vi "Add data or replace.vi"(9 "Power data":cluster{"Frequency (GHz)":dbl, "Power (mW)":dbl}, 10 "Index":i32, 11 "Power readings in":cluster{"Frequency":dbl, "Power":dbl}[](array[cluster])) -> (3 "Power readings out":cluster{"Frequency":dbl, "Power":dbl}[](array[cluster]))   [LabVIEW 2019, in "Power control.lvclass"]
uses:
  Power control.lvclass
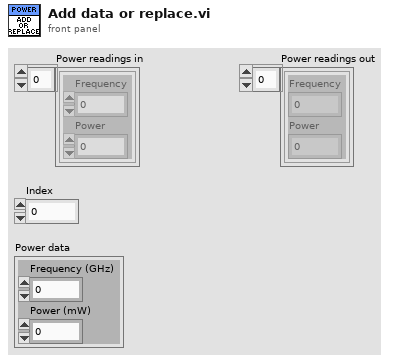
[diagram p1: front panel]
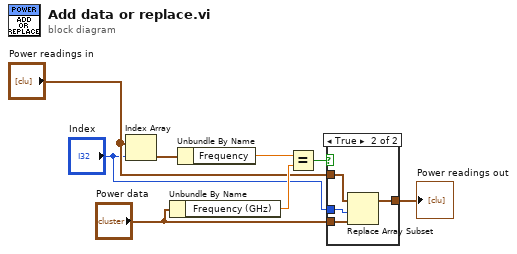
[diagram p0: block diagram]
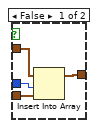
[diagram p2: hidden frame]
diagram:
  n1 = Index Array(array="Power readings in", index="Index") -> (element=w3:cluster{"Frequency":dbl, "Power":dbl})
  n2 = Unbundle By Name("Power data") -> ("Frequency (GHz)"=w6:dbl)
  n3 = Unbundle By Name(w3) -> ("Frequency"=w2:dbl)
  n4 = Equal?(x=w2, y=w6) -> (x = y?=w1:bool)
  n5 = case shown="True" w1 {
    tunnel: "Power data" -> [w12 w14]
    tunnel: "Index" -> [w11 w15]
    tunnel: [w10 w13] -> w8
    tunnel: "Power readings in" -> [w9 w16]
    frame False {
      n6 = Insert Into Array(array=w9, index=w11, new element=w12) -> (w10:cluster{"Frequency":dbl, "Power":dbl}[])
    }
    frame True {
      n7 = Replace Array Subset(array=w16, new element=w14, index=w15) -> (w13:cluster{"Frequency":dbl, "Power":dbl}[])
    }
  }
  "Power readings out" <- w8
